vi "List Mapped Keys.vi"(8 "error in (no error)":errorcluster, 11 "JobReport in":refnum<class "JobReport.lvclass">) -> (0 "error out":errorcluster, 2 "Mapped Keys":string[](array[string]), 3 "JobReport out":refnum<class "JobReport.lvclass">)   [LabVIEW 2013, in "openCronJob.lvlib" / "JobReport.lvclass"]
uses:
  JobReport.lvclass
  JobReport.lvclass/JobReport.ctl
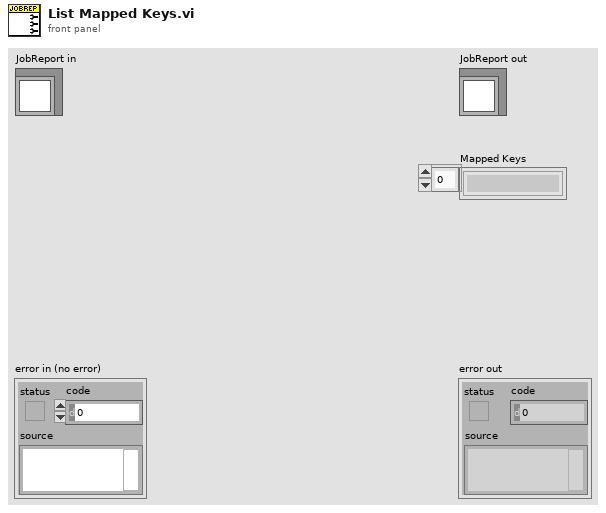
[diagram p1: front panel]
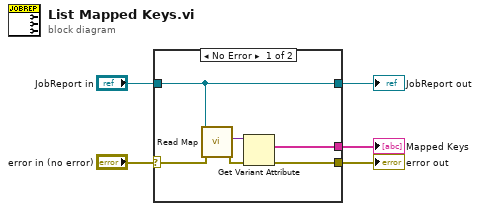
[diagram p0: block diagram]
diagram:
  n1 = case shown="No Error" "error in (no error)" {
    selector: "error in (no error)" -> [w7 w13]
    tunnel: [w6 w13] -> w4
    tunnel: [w11 w12] -> w2
    tunnel: "JobReport in" -> [w11 w12]
    tunnel: [w9 _] -> w1
    frame No Error {
      n2 = call "Read Map.vi"("error in (no error)"=w7, "JobReport in"=w11) -> ("error out"=w8:errorcluster, "Map"=w10:variant)  [unwired: 7 in, 1 out]
      n3 = Get Variant Attribute(Variant=w10, error in=w8) -> (names=w9:string[], error out=w6:errorcluster)  [unwired: 2 in, 2 out]
    }
    frame Error {
    }
  }
  "error out" <- w4
  "JobReport out" <- w2
  "Mapped Keys" <- w1
